vi "Run Post-Hook.vi"(8 "Error In":errorcluster, 10 "Writer In":refnum<class "Writer.lvclass">, 11 "Context In":refnum<class "Compiler.lvclass">) -> (0 "Error Out":errorcluster, 2 "Writer Out":refnum<class "Writer.lvclass">, 3 "Context Out":refnum<class "Compiler.lvclass">)   [LabVIEW 2018, in "Toolkit.lvlib" / "Renderer.lvclass"]
uses:
  Renderer.lvclass
  Hooks/Render/Process/Process.lvclass
  Compiler/Compiler.lvclass
  Data/Datum/Datum.lvclass
  D:/Users/cfield/Code/Field R&D Services/Labstache/src/Toolkit/Hooks/Hook/Hook.lvclass
  Writers/Writer/Writer.lvclass
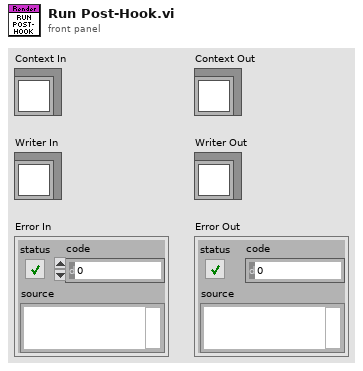
[diagram p1: front panel]
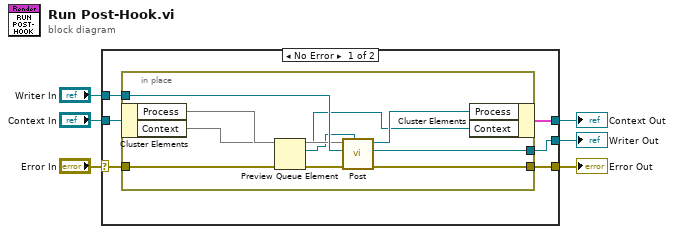
[diagram p0: block diagram]
diagram:
  n1 = case shown="No Error" "Error In" {
    selector: "Error In" -> [w9 w24]
    tunnel: [w12 w25] -> w6
    tunnel: "Writer In" -> [w11 w25]
    tunnel: [w10 w24] -> w4
    tunnel: "Context In" -> [w8 w23]
    tunnel: [w7 w23] -> w1
    frame No Error {
      n2 = in-place {
        in-place-border: [w22] -> w12
        in-place-border: w11 -> [w21]
        in-place-border: [w20] -> w10
        in-place-border: w9 -> [w19]
        n3 = in-place-cluster #1(w8) -> ("Process"=w18, "Context"=w15)
        n4 = Preview Queue Element(queue=w15, error in (no error)=w19) -> (queue out=w14:refnum<queue>, element=w13:refnum<class "Datum.lvclass">, error out=w16:errorcluster)  [unwired: 1 in, 1 out]
        n5 = call-dynamic "Post.vi"("Datum"=w13, "Error In"=w16, "Writer In"=w21, "Render In"=w18) -> ("Error Out"=w20:errorcluster, "Writer Out"=w22:refnum<class "Writer.lvclass">, "Render Out"=w17:refnum<class "Process.lvclass">)  [unwired: 5 in]
        n6 = in-place-cluster #1("Process"=w17, "Context"=w14) -> (w7:cluster{})
      }
    }
    frame Error {
    }
  }
  "Writer Out" <- w6
  "Error Out" <- w4
  "Context Out" <- w1
